vi "Config_File_Parser.vi"() -> ()   [LabVIEW 2018]
uses:
  <vilib>/xml/Load XML File.vi
  <vilib>/xml/Close Reference(Node).vi
  <vilib>/xml/NI_XML.lvlib
  <resource>/objmgr/DOMUserDefRef.rc
panel:
  in  "stop":bool
  out "Program":string[][](array[string])
  out "Positions":dbl[][](array[numeric])
  out "Filter":string[][](array[string])
  out "Objective":string[](array[string])
  out "Prism Loop":string
  out "SOLA":string
  out "Pressure Loop":dbl[](array[numeric])
  out "SaveDir":string
  out "Aquisition Interval":string
  out "Image Prefix":string
  out "Duration":string
  out "Pressure":dbl[](array[numeric])
  out "Lamp":string
  out "Prism":string
  out "Filter":string
  out "Objective":string
  out "XML":string
  out "Parse Errors":string
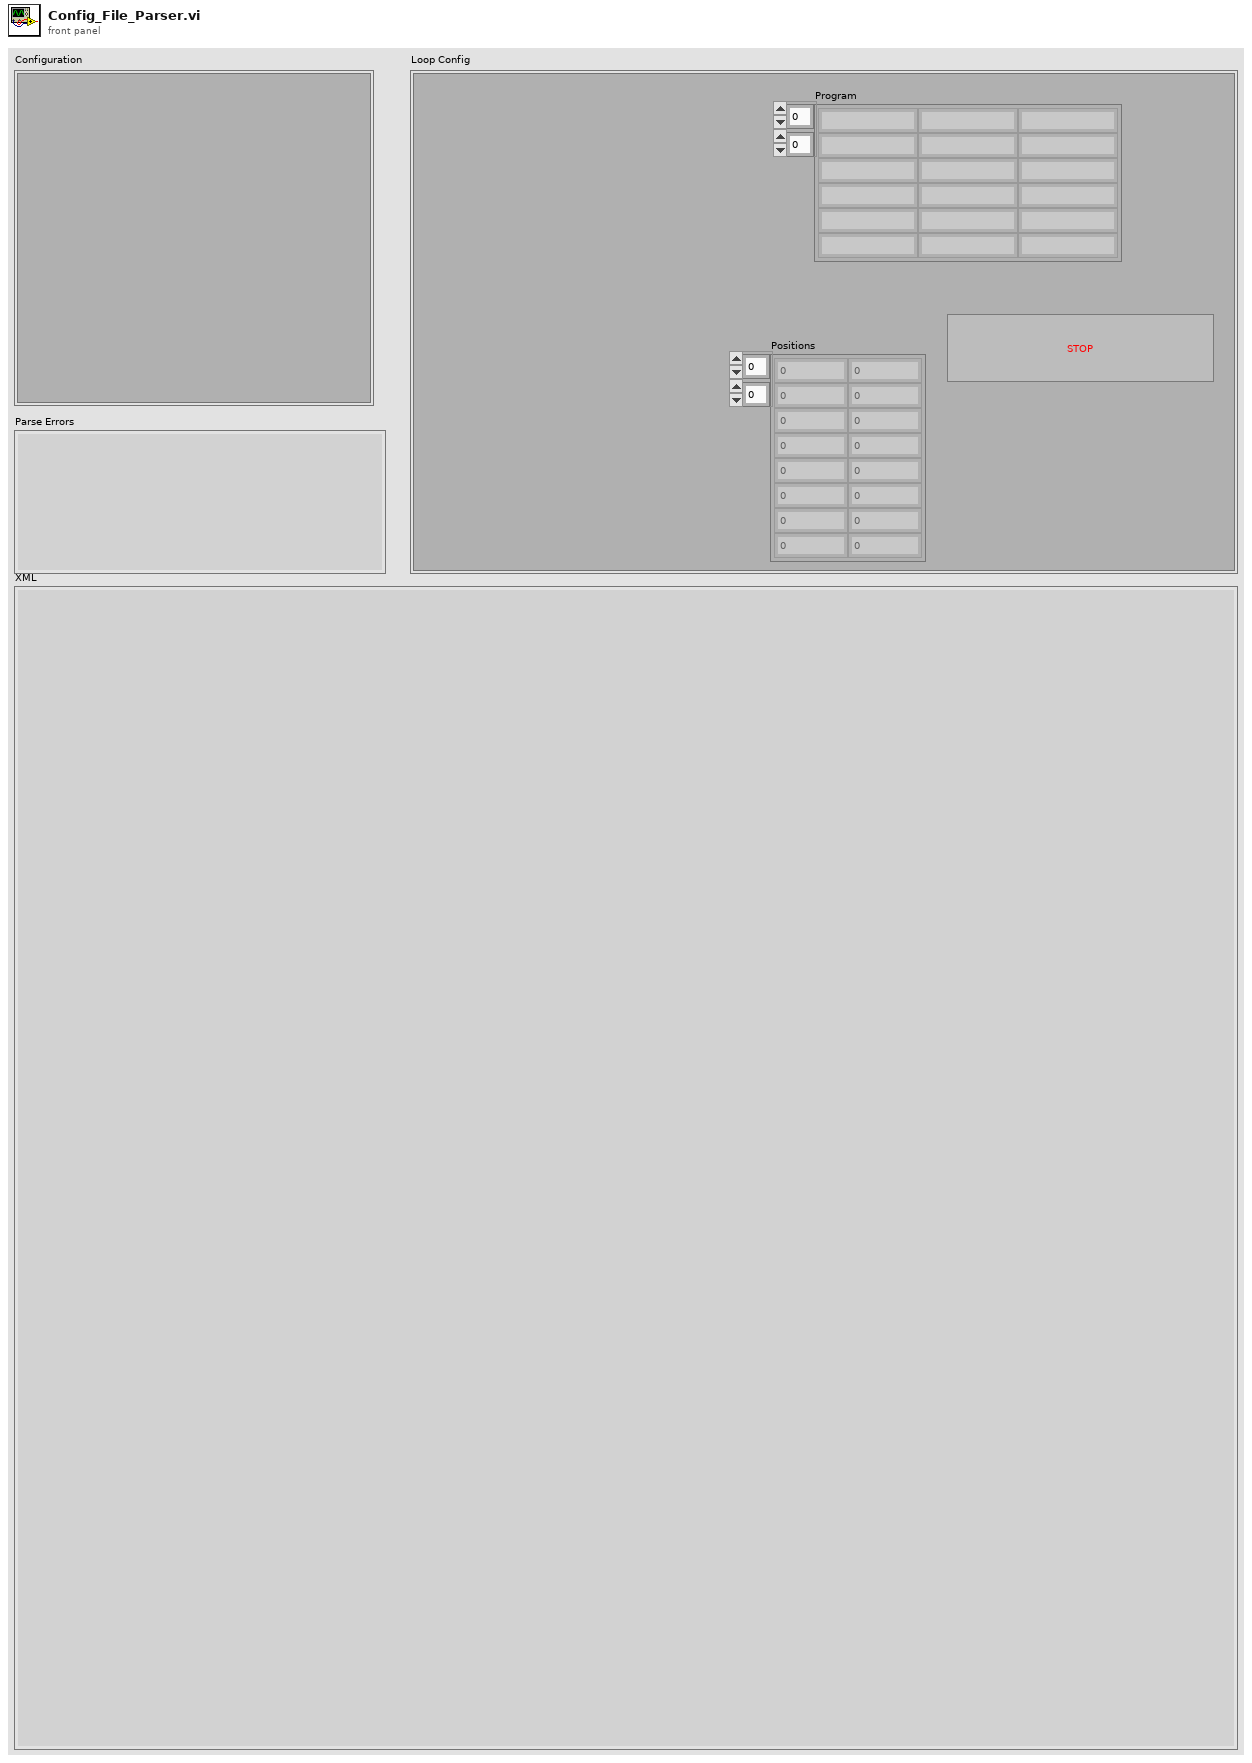
[diagram p1: front panel]
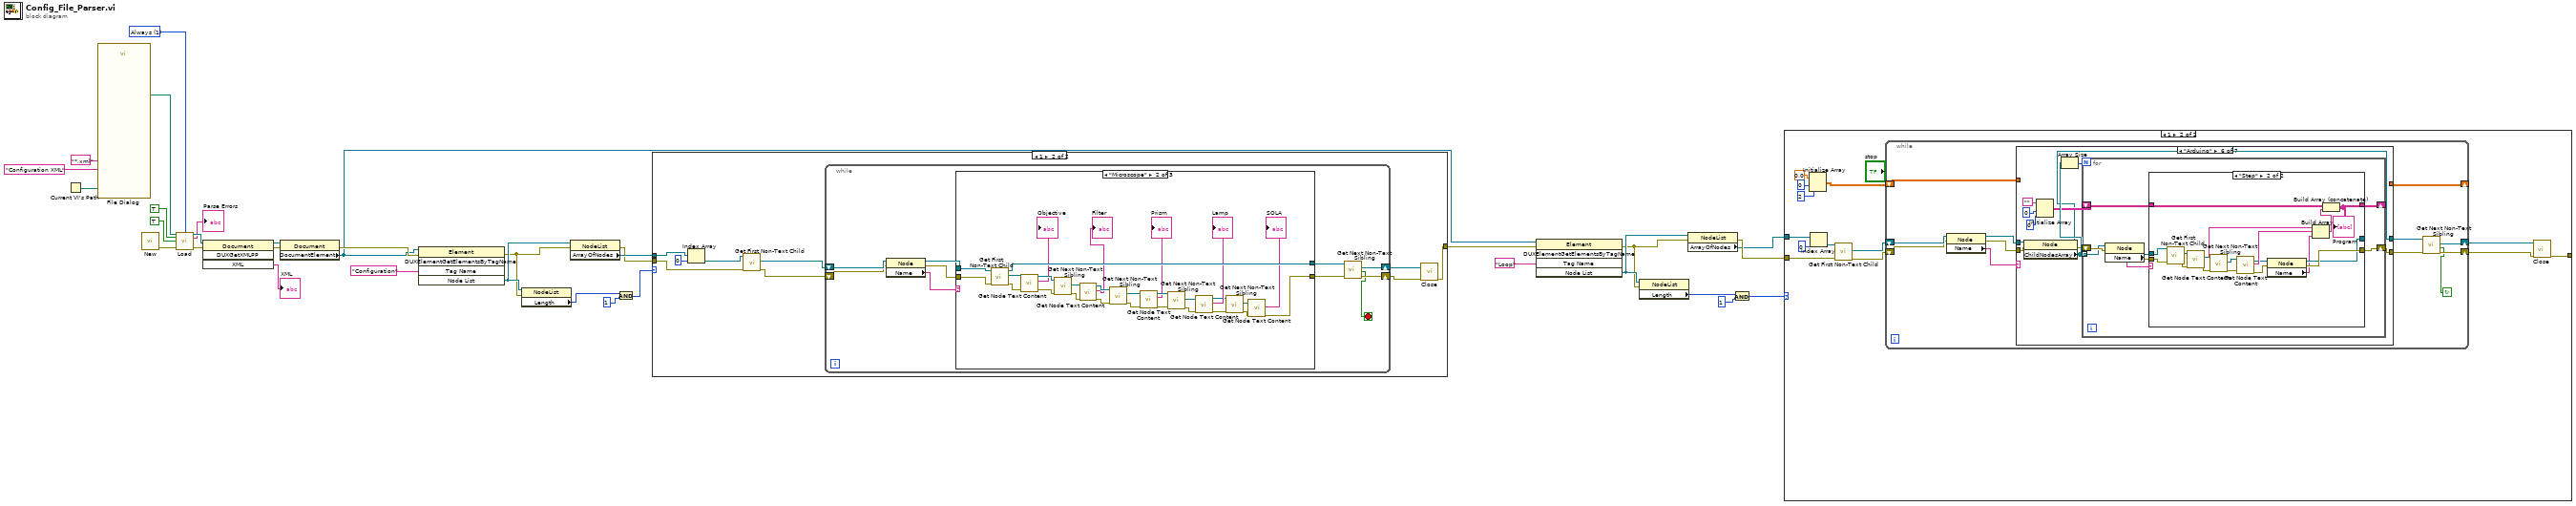
[diagram p0: block diagram]
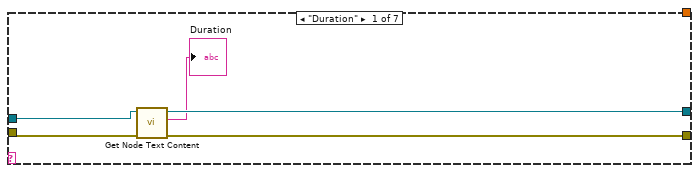
[diagram p3: hidden frame]
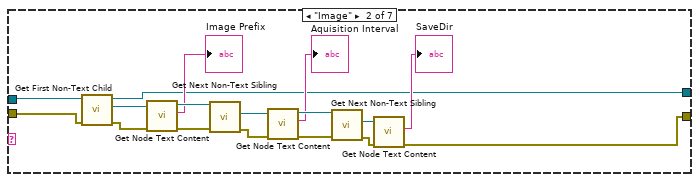
[diagram p4: hidden frame]
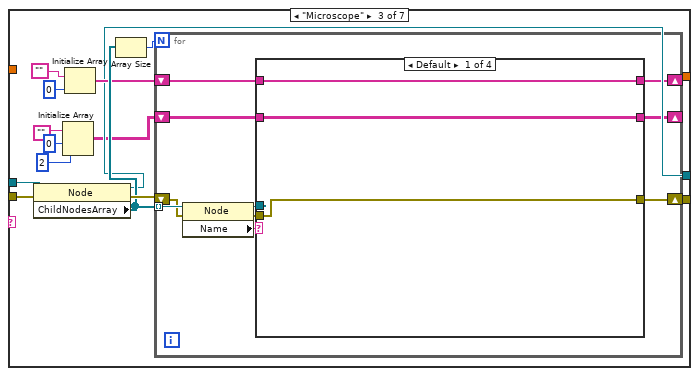
[diagram p5: hidden frame]
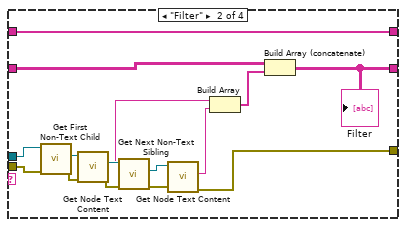
[diagram p6: hidden frame]
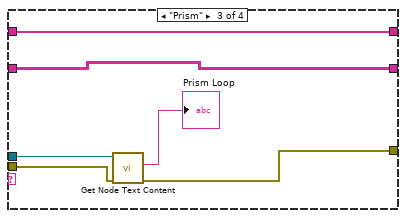
[diagram p7: hidden frame]
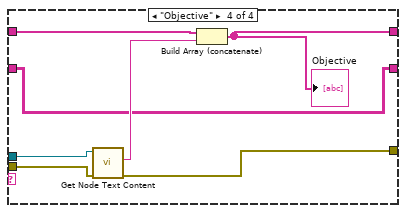
[diagram p8: hidden frame]
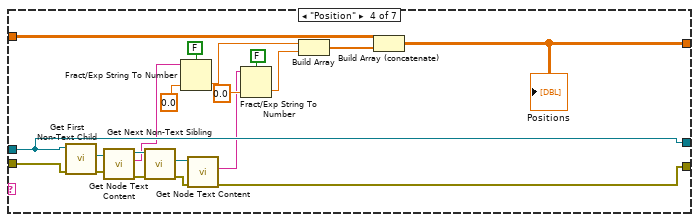
[diagram p9: hidden frame]
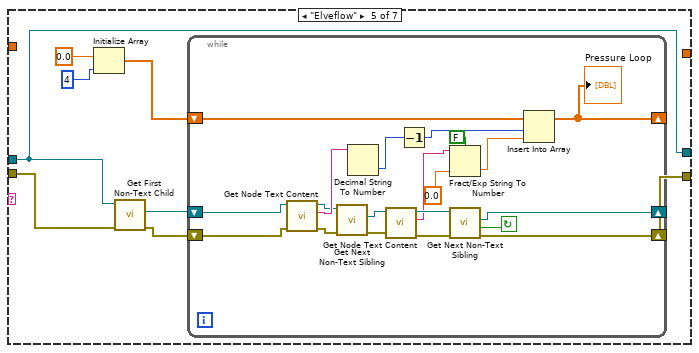
[diagram p10: hidden frame]
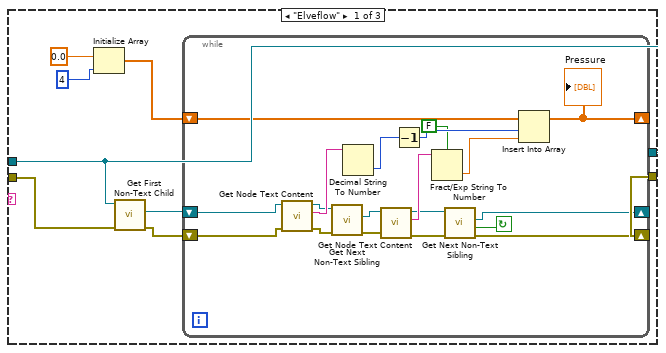
[diagram p14: hidden frame]
diagram:
  w23 = 1 items=["Never", "Always", "Auto"] ("validate on load (Auto)")
  n1 = Current VI's Path() -> (path=w31:path)
  n2 = call "File Dialog"("start path"=w31, "pattern (all files)"="*.xml", "pattern label"="Configuration XML") -> ("selected path"=w28:path)  [unwired: 9 in, 3 out]
  n3 = call <vilib>:"New.vi"() -> ("error out"=w29:errorcluster)  [unwired: 8 in, 1 out]
  n4 = call-poly <vilib>:"Load.vi"("path to XML document"=w28, "validate on load (Auto)"=w23, "process namespaces (False)"=TRUE, "process schema (False)"=TRUE, "error in (no error)"=w29) -> ("DOM document out"=w26:refnum<k20>, "parse errors"=→"Parse Errors":string, "error out"=w25:errorcluster)  [unwired: 8 in]
  n5 = invoke class="Document" method="DUXGetXMLPP"(reference=w26, error in=w25) -> (reference out=w21:refnum<k20>, error out=w20:errorcluster, "XML"=→"XML":string)  [unwired: 2 in, 1 out]
  n6 = property class="Document"(reference=w21, error in=w20) -> (error out=w19:errorcluster, "DocumentElement"=w5:refnum<k20>)  [unwired: 1 out]
  n7 = invoke class="Element" method="DUXElementGetElementsByTagName"(reference=w5, error in=w19, "Tag Name"="Configuration" ("Get Elements By Tag Name")) -> (error out=w13:errorcluster, "Node List"=w14:refnum<k20>)  [unwired: 2 in, 3 out]
  n8 = property class="NodeList"(reference=w14, error in=w13) -> ("Length"=w15:i32)  [unwired: 2 out]
  n9 = property class="NodeList"(reference=w14, error in=w13) -> (error out=w11:errorcluster, "ArrayOfNodes"=w12:refnum<k20>[])  [unwired: 1 out]
  n10 = And(x=w15, y=1) -> (x .and. y?=w16:i32)
  n11 = case shown="1" w16 {
    tunnel: w12 -> [_ w43]
    tunnel: w11 -> [w34 w38]
    tunnel: [w34 w35] -> w4
    frame 0, Default {
    }
    frame 1 {
      n12 = Index Array(array=w43, index=0) -> (element=w39:refnum<k20>)
      n13 = call <vilib>:"Get First Non-Text Child.vi"("error in (no error)"=w38, "node in"=w39) -> ("error out"=w40:errorcluster, "child node"=w41:refnum<k20>)  [unwired: 6 in, 2 out]
      n14 = while {
        shift-right: [w47] -> w37
        shift-left: w41 -> [w50]
        shift-right: [w48] -> w36
        shift-left: w40 -> [w49]
        stop <- w46 stop-if-true
        n15 = property class="Node"(reference=w50, error in=w49) -> (reference out=w53:refnum<k20>, error out=w52:errorcluster, "Name"=w51:string)
        n16 = case shown="\"Microscope\"" w51 {
          tunnel: w52 -> [w58 w106 w109]
          tunnel: w53 -> [w59 w107 w108]
          tunnel: [w59 w91 w108] -> w45
          tunnel: [w55 w81 w109] -> w44
          frame "Elveflow" {
            n17 = Initialize Array(0.0, 4) -> (w54:dbl[])
            n18 = call <vilib>:"Get First Non-Text Child.vi"("error in (no error)"=w58, "node in"=w59) -> ("error out"=w56:errorcluster, "child node"=w57:refnum<k20>)  [unwired: 6 in, 2 out]
            n19 = while {
              shift-right: [w69] -> w55
              shift-left: w56 -> [w73]
              shift-right: [w70] -> _
              shift-left: w57 -> [w74]
              shift-right: [w63] -> _
              shift-left: w54 -> [w68]
              stop <- w67 continue-if-true
              n20 = call <vilib>:"Get Node Text Content.vi"("error in (no error)"=w73, "node in"=w74) -> ("error out"=w75:errorcluster, "node text"=w78:string, "node out"=w76:refnum<k20>)  [unwired: 7 in]
              n21 = call <vilib>:"Get Next Non-Text Sibling.vi"("error in (no error)"=w75, "node in"=w76) -> ("error out"=w77:errorcluster, "sibling node"=w66:refnum<k20>)  [unwired: 6 in, 2 out]
              n22 = Decimal String To Number(string=w78) -> (number=w65:i32)  [unwired: 2 in, 1 out]
              n23 = call <vilib>:"Get Node Text Content.vi"("error in (no error)"=w77, "node in"=w66) -> ("error out"=w71:errorcluster, "node text"=w79:string, "node out"=w72:refnum<k20>)  [unwired: 7 in]
              n24 = Decrement(x=w65) -> (x-1=w64:i32)
              n25 = Fract/Exp String To Number(use system decimal point (T)=FALSE, string=w79) -> (number=w80:dbl)  [unwired: 2 in, 1 out]
              n26 = call <vilib>:"Get Next Non-Text Sibling.vi"("error in (no error)"=w71, "node in"=w72) -> ("error out"=w69:errorcluster, "found sibling node?"=w67:bool, "sibling node"=w70:refnum<k20>)  [unwired: 6 in, 1 out]
              n27 = Insert Into Array(array=w68, index=w64, new element=w80) -> (w63:dbl[])
              "Pressure" <- w63
            }
          }
          frame "Microscope" {
            n28 = call <vilib>:"Get First Non-Text Child.vi"("error in (no error)"=w106, "node in"=w107) -> ("error out"=w105:errorcluster, "child node"=w104:refnum<k20>, "node out"=w91:refnum<k20>)  [unwired: 6 in, 1 out]
            n29 = call <vilib>:"Get Node Text Content.vi"("error in (no error)"=w105, "node in"=w104) -> ("error out"=w102:errorcluster, "node text"=→"Objective":string, "node out"=w103:refnum<k20>)  [unwired: 7 in]
            n30 = call <vilib>:"Get Next Non-Text Sibling.vi"("error in (no error)"=w102, "node in"=w103) -> ("error out"=w101:errorcluster, "sibling node"=w100:refnum<k20>)  [unwired: 6 in, 2 out]
            n31 = call <vilib>:"Get Node Text Content.vi"("error in (no error)"=w101, "node in"=w100) -> ("error out"=w99:errorcluster, "node text"=→"Filter":string, "node out"=w98:refnum<k20>)  [unwired: 7 in]
            n32 = call <vilib>:"Get Next Non-Text Sibling.vi"("error in (no error)"=w99, "node in"=w98) -> ("error out"=w97:errorcluster, "sibling node"=w96:refnum<k20>)  [unwired: 6 in, 2 out]
            n33 = call <vilib>:"Get Node Text Content.vi"("error in (no error)"=w97, "node in"=w96) -> ("error out"=w95:errorcluster, "node text"=→"Prism":string, "node out"=w94:refnum<k20>)  [unwired: 7 in]
            n34 = call <vilib>:"Get Next Non-Text Sibling.vi"("error in (no error)"=w95, "node in"=w94) -> ("error out"=w93:errorcluster, "sibling node"=w92:refnum<k20>)  [unwired: 6 in, 2 out]
            n35 = call <vilib>:"Get Node Text Content.vi"("error in (no error)"=w93, "node in"=w92) -> ("error out"=w84:errorcluster, "node text"=→"Lamp":string, "node out"=w85:refnum<k20>)  [unwired: 7 in]
            n36 = call <vilib>:"Get Next Non-Text Sibling.vi"("error in (no error)"=w84, "node in"=w85) -> ("error out"=w82:errorcluster, "sibling node"=w83:refnum<k20>)  [unwired: 6 in, 2 out]
            n37 = call <vilib>:"Get Node Text Content.vi"("error in (no error)"=w82, "node in"=w83) -> ("error out"=w81:errorcluster, "node text"=→"SOLA":string)  [unwired: 7 in, 1 out]
          }
          frame Default {
          }
        }
        n38 = call <vilib>:"Get Next Non-Text Sibling.vi"("error in (no error)"=w44, "node in"=w45) -> ("error out"=w48:errorcluster, "found sibling node?"=w46:bool, "sibling node"=w47:refnum<k20>)  [unwired: 6 in, 1 out]
      }
      n39 = call-poly <vilib>:"Close.vi"("error in (no error)"=w36, "node"=w37) -> ("error out"=w35:errorcluster)  [unwired: 7 in]
    }
  }
  n40 = invoke class="Element" method="DUXElementGetElementsByTagName"(reference=w5, error in=w4, "Tag Name"="Loop" ("Get Elements By Tag Name")) -> (error out=w6:errorcluster, "Node List"=w7:refnum<k20>)  [unwired: 2 in, 3 out]
  n41 = property class="NodeList"(reference=w7, error in=w6) -> ("Length"=w8:i32)  [unwired: 2 out]
  n42 = property class="NodeList"(reference=w7, error in=w6) -> (error out=w2:errorcluster, "ArrayOfNodes"=w1:refnum<k20>[])  [unwired: 1 out]
  n43 = And(x=w8, y=1) -> (x .and. y?=w3:i32)
  n44 = case shown="1" w3 {
    tunnel: w2 -> [w110 w120]
    tunnel: w1 -> [_ w121]
    tunnel: [w110 w117] -> _
    frame 0, Default {
    }
    frame 1 {
      n45 = Initialize Array(0.0 ("element"), 0 ("dimension size"), 2 ("dimension size")) -> (w111:dbl[][])
      n46 = Index Array(array=w121, index=0) -> (element=w123:refnum<k20>)
      n47 = call <vilib>:"Get First Non-Text Child.vi"("error in (no error)"=w120, "node in"=w123) -> ("error out"=w118:errorcluster, "child node"=w119:refnum<k20>)  [unwired: 6 in, 2 out]
      n48 = while {
        shift-right: [w130] -> w115
        shift-left: w119 -> [w133]
        shift-right: [w131] -> w116
        shift-left: w118 -> [w132]
        shift-right: [w126] -> _
        shift-left: w111 -> [w125]
        stop <- w129 continue-if-true
        n49 = property class="Node"(reference=w133, error in=w132) -> (reference out=w135:refnum<k20>, error out=w124:errorcluster, "Name"=w134:string)
        n50 = case shown="\"Arduino\"" w134 {
          tunnel: w124 -> [w139 w148 w170 w232 w238 w271 w303]
          tunnel: w135 -> [w140 w149 w171 w222 w233 w270 w302]
          tunnel: [w138 w141 w161 w222 w233 w262 w302] -> w128
          tunnel: [w137 w142 w162 w221 w235 w267 w303] -> w127
          tunnel: w125 -> [_ _ _ w224 _ _ w301]
          tunnel: [_ _ _ w223 _ _ w301] -> w126
          frame "Duration" {
            n51 = call <vilib>:"Get Node Text Content.vi"("error in (no error)"=w139, "node in"=w140) -> ("error out"=w137:errorcluster, "node text"=→"Duration":string, "node out"=w138:refnum<k20>)  [unwired: 7 in]
          }
          frame "Image" {
            n52 = call <vilib>:"Get First Non-Text Child.vi"("error in (no error)"=w148, "node in"=w149) -> ("error out"=w150:errorcluster, "child node"=w151:refnum<k20>, "node out"=w141:refnum<k20>)  [unwired: 6 in, 1 out]
            n53 = call <vilib>:"Get Node Text Content.vi"("error in (no error)"=w150, "node in"=w151) -> ("error out"=w153:errorcluster, "node text"=→"Image Prefix":string, "node out"=w152:refnum<k20>)  [unwired: 7 in]
            n54 = call <vilib>:"Get Next Non-Text Sibling.vi"("error in (no error)"=w153, "node in"=w152) -> ("error out"=w154:errorcluster, "sibling node"=w155:refnum<k20>)  [unwired: 6 in, 2 out]
            n55 = call <vilib>:"Get Node Text Content.vi"("error in (no error)"=w154, "node in"=w155) -> ("error out"=w156:errorcluster, "node text"=→"Aquisition Interval":string, "node out"=w157:refnum<k20>)  [unwired: 7 in]
            n56 = call <vilib>:"Get Next Non-Text Sibling.vi"("error in (no error)"=w156, "node in"=w157) -> ("error out"=w144:errorcluster, "sibling node"=w145:refnum<k20>)  [unwired: 6 in, 2 out]
            n57 = call <vilib>:"Get Node Text Content.vi"("error in (no error)"=w144, "node in"=w145) -> ("error out"=w142:errorcluster, "node text"=→"SaveDir":string)  [unwired: 7 in, 1 out]
          }
          frame "Microscope" {
            n58 = property class="Node"(reference=w171, error in=w170) -> (reference out=w161:refnum<k20>, error out=w168:errorcluster, "ChildNodesArray"=w167:refnum<k20>[])
            n59 = Initialize Array("", 0 ("dimension size"), 2 ("dimension size")) -> (w158:string[][])
            n60 = Initialize Array("", 0 ("dimension size")) -> (w165:string[])
            n61 = Array Size(array=w167) -> (size(s)=w169:i32)
            n62 = for {
              N: w169 -> [_]
              tunnel: w167 -> [w181] mode=indexing
              shift-right: [w173] -> _
              shift-left: w165 -> [w174]
              shift-right: [w176] -> w162
              shift-left: w168 -> [w180]
              shift-right: [w172] -> _
              shift-left: w158 -> [w175]
              n63 = property class="Node"(reference=w181, error in=w180) -> (reference out=w179:refnum<k20>, error out=w178:errorcluster, "Name"=w177:string)
              n64 = case shown="Default" w177 {
                tunnel: w179 -> [_ w191 w205 w212]
                tunnel: w178 -> [w182 w190 w204 w211]
                tunnel: w174 -> [w184 w185 w201 w210]
                tunnel: [w182 w186 w202 w207] -> w176
                tunnel: w175 -> [w183 w199 w200 w206]
                tunnel: [w184 w185 w201 w208] -> w173
                tunnel: [w183 w198 w200 w206] -> w172
                frame Default {
                }
                frame "Filter" {
                  n65 = call <vilib>:"Get First Non-Text Child.vi"("error in (no error)"=w190, "node in"=w191) -> ("error out"=w193:errorcluster, "child node"=w192:refnum<k20>)  [unwired: 6 in, 2 out]
                  n66 = call <vilib>:"Get Node Text Content.vi"("error in (no error)"=w193, "node in"=w192) -> ("error out"=w195:errorcluster, "node text"=w189:string, "node out"=w196:refnum<k20>)  [unwired: 7 in]
                  n67 = call <vilib>:"Get Next Non-Text Sibling.vi"("error in (no error)"=w195, "node in"=w196) -> ("error out"=w197:errorcluster, "sibling node"=w194:refnum<k20>)  [unwired: 6 in, 2 out]
                  n68 = call <vilib>:"Get Node Text Content.vi"("error in (no error)"=w197, "node in"=w194) -> ("error out"=w186:errorcluster, "node text"=w188:string)  [unwired: 7 in, 1 out]
                  n69 = Build Array(w189, w188) -> (w187:string[])
                  n70 = Build Array (concatenate)(w199, w187) -> (w198:string[][])
                  "Filter" <- w198
                }
                frame "Prism" {
                  n71 = call <vilib>:"Get Node Text Content.vi"("error in (no error)"=w204, "node in"=w205) -> ("error out"=w202:errorcluster, "node text"=→"Prism Loop":string)  [unwired: 7 in, 1 out]
                }
                frame "Objective" {
                  n72 = call <vilib>:"Get Node Text Content.vi"("error in (no error)"=w211, "node in"=w212) -> ("error out"=w207:errorcluster, "node text"=w209:string)  [unwired: 7 in, 1 out]
                  n73 = Build Array (concatenate)(w210, w209) -> (w208:string[])
                  "Objective" <- w208
                }
              }
            }
          }
          frame "Position" {
            n74 = call <vilib>:"Get First Non-Text Child.vi"("error in (no error)"=w232, "node in"=w222) -> ("error out"=w231:errorcluster, "child node"=w230:refnum<k20>)  [unwired: 6 in, 2 out]
            n75 = call <vilib>:"Get Node Text Content.vi"("error in (no error)"=w231, "node in"=w230) -> ("error out"=w229:errorcluster, "node text"=w219:string, "node out"=w228:refnum<k20>)  [unwired: 7 in]
            n76 = call <vilib>:"Get Next Non-Text Sibling.vi"("error in (no error)"=w229, "node in"=w228) -> ("error out"=w227:errorcluster, "sibling node"=w226:refnum<k20>)  [unwired: 6 in, 2 out]
            n77 = Fract/Exp String To Number(use system decimal point (T)=FALSE, string=w219, default (0 dbl)=0.0 ("default (0 I32)")) -> (number=w215:dbl)  [unwired: 1 in, 1 out]
            n78 = call <vilib>:"Get Node Text Content.vi"("error in (no error)"=w227, "node in"=w226) -> ("error out"=w221:errorcluster, "node text"=w217:string)  [unwired: 7 in, 1 out]
            n79 = Fract/Exp String To Number(use system decimal point (T)=FALSE, string=w217, default (0 dbl)=0.0 ("default (0 I32)")) -> (number=w216:dbl)  [unwired: 1 in, 1 out]
            n80 = Build Array(w215, w216) -> (w225:dbl[])
            n81 = Build Array (concatenate)(w224, w225) -> (w223:dbl[][])
            "Positions" <- w223
          }
          frame "Elveflow" {
            n82 = Initialize Array(0.0, 4) -> (w234:dbl[])
            n83 = call <vilib>:"Get First Non-Text Child.vi"("error in (no error)"=w238, "node in"=w233) -> ("error out"=w236:errorcluster, "child node"=w237:refnum<k20>)  [unwired: 6 in, 2 out]
            n84 = while {
              shift-right: [w251] -> w235
              shift-left: w236 -> [w255]
              shift-right: [w252] -> _
              shift-left: w237 -> [w256]
              shift-right: [w245] -> _
              shift-left: w234 -> [w250]
              stop <- w249 continue-if-true
              n85 = call <vilib>:"Get Node Text Content.vi"("error in (no error)"=w255, "node in"=w256) -> ("error out"=w257:errorcluster, "node text"=w260:string, "node out"=w258:refnum<k20>)  [unwired: 7 in]
              n86 = call <vilib>:"Get Next Non-Text Sibling.vi"("error in (no error)"=w257, "node in"=w258) -> ("error out"=w259:errorcluster, "sibling node"=w248:refnum<k20>)  [unwired: 6 in, 2 out]
              n87 = Decimal String To Number(string=w260) -> (number=w247:i32)  [unwired: 2 in, 1 out]
              n88 = call <vilib>:"Get Node Text Content.vi"("error in (no error)"=w259, "node in"=w248) -> ("error out"=w253:errorcluster, "node text"=w244:string, "node out"=w254:refnum<k20>)  [unwired: 7 in]
              n89 = Decrement(x=w247) -> (x-1=w246:i32)
              n90 = Fract/Exp String To Number(use system decimal point (T)=FALSE, string=w244, default (0 dbl)=0.0 ("default (0 I32)")) -> (number=w242:dbl)  [unwired: 1 in, 1 out]
              n91 = call <vilib>:"Get Next Non-Text Sibling.vi"("error in (no error)"=w253, "node in"=w254) -> ("error out"=w251:errorcluster, "found sibling node?"=w249:bool, "sibling node"=w252:refnum<k20>)  [unwired: 6 in, 1 out]
              n92 = Insert Into Array(array=w250, index=w246, new element=w242) -> (w245:dbl[])
              "Pressure Loop" <- w245
            }
          }
          frame "Arduino" {
            n93 = property class="Node"(reference=w270, error in=w271) -> (reference out=w262:refnum<k20>, error out=w261:errorcluster, "ChildNodesArray"=w268:refnum<k20>[])
            n94 = Initialize Array("", 0 ("dimension size"), 0 ("dimension size")) -> (w266:string[][])
            n95 = Array Size(array=w268) -> (size(s)=w269:i32)
            n96 = for {
              N: w269 -> [_]
              shift-right: [w276] -> w267
              shift-left: w261 -> [w273]
              shift-right: [w274] -> _
              shift-left: w266 -> [w275]
              tunnel: w268 -> [w272] mode=indexing
              n97 = property class="Node"(reference=w272, error in=w273) -> (reference out=w279:refnum<k20>, error out=w278:errorcluster, "Name"=w277:string)
              n98 = case shown="\"Step\"" w277 {
                tunnel: w279 -> [w280 w292]
                tunnel: w278 -> [w281 w291]
                tunnel: [w281 w285] -> w276
                tunnel: w275 -> [w282 w300]
                tunnel: [w282 w299] -> w274
                tunnel: [w280 w284] -> _
                frame Default {
                }
                frame "Step" {
                  n99 = call <vilib>:"Get First Non-Text Child.vi"("error in (no error)"=w291, "node in"=w292) -> ("error out"=w294:errorcluster, "child node"=w293:refnum<k20>)  [unwired: 6 in, 2 out]
                  n100 = call <vilib>:"Get Node Text Content.vi"("error in (no error)"=w294, "node in"=w293) -> ("error out"=w296:errorcluster, "node text"=w290:string, "node out"=w297:refnum<k20>)  [unwired: 7 in]
                  n101 = call <vilib>:"Get Next Non-Text Sibling.vi"("error in (no error)"=w296, "node in"=w297) -> ("error out"=w298:errorcluster, "sibling node"=w295:refnum<k20>)  [unwired: 6 in, 2 out]
                  n102 = call <vilib>:"Get Node Text Content.vi"("error in (no error)"=w298, "node in"=w295) -> ("error out"=w286:errorcluster, "node text"=w289:string, "node out"=w287:refnum<k20>)  [unwired: 7 in]
                  n103 = property class="Node"(reference=w287, error in=w286) -> (reference out=w284:refnum<k20>, error out=w285:errorcluster, "Name"=w283:string)
                  n104 = Build Array(w290, w289, w283) -> (w288:string[])
                  n105 = Build Array (concatenate)(w300, w288) -> (w299:string[][])
                  "Program" <- w299
                }
              }
            }
          }
          frame Default {
          }
        }
        n106 = call <vilib>:"Get Next Non-Text Sibling.vi"("error in (no error)"=w127, "node in"=w128) -> ("error out"=w131:errorcluster, "found sibling node?"=w129:bool, "sibling node"=w130:refnum<k20>)  [unwired: 6 in, 1 out]
      }
      n107 = call-poly <vilib>:"Close.vi"("error in (no error)"=w116, "node"=w115) -> ("error out"=w117:errorcluster)  [unwired: 7 in]
    }
  }
